vi "Facade.vi"(0 "Data In":T7, 2 "Display State In":T4, 3 "Container State":T6) -> (6 "Data Out":T7, 7 "Display State Out":T4, 8 "Action":T3)   [LabVIEW 2017, in "2D Feather.xctl"]
uses:
  <vilib>/Math Plots/2D Math Plots/2D Feather/2D Feather XCtrl/2D Feather.xctl
  <vilib>/Math Plots/2D Math Plots/2D Feather/2D Feather XCtrl/Data.ctl
  <vilib>/Math Plots/2D Math Plots/2D Plot/2D Plot Datatype/2D Plot Datatype.lvclass
  <vilib>/_xctls/Container State.ctl
  <vilib>/Math Plots/2D Math Plots/2D Feather/2D Feather XCtrl/State.ctl
  <vilib>/Math Plots/2D Math Plots/2D Feather/2D Feather/2D Feather.lvclass
  e:/builds/penguin/labview/branches/2017/dev/dist/vi.lib/Math Plots/2D Math Plots/2D Plot/2D Plot/2D Plot.lvclass
  <vilib>/Math Plots/2D Math Plots/2D Plot/Action String/2DMathPlot Ctrl Act Queue.ctl
  <vilib>/Math Plots/2D Math Plots/2D Plot/Action String/2DMathPlot Ctrl Act Cluster.ctl
  <vilib>/Math Plots/2D Math Plots/2D Plot/Action String/2DMathPlot State Class.ctl
  <vilib>/_xctls/Action.ctl
  <vilib>/Math Plots/2D Math Plots/2D Plot/2D Plot/Typedef/Range Cluster.ctl
  <vilib>/Math Plots/2D Math Plots/2D Plot/Action String/2DMathPlot Action String.ctl
  <vilib>/_xctls/XControlSupport.lvlib
  <vilib>/Math Plots/2D Math Plots/2D Plot/2D Plot/2D Plot.lvclass
panel:
  out "Floating":string
  in  "Customized Plot Legend":T1={"Color Pair Array"=[{"String"="Plot 0", "Picture"=bytes[184]}, {"String"="Plot 2", "Picture"=bytes[92]}, {"String"="Plot 3", "Picture"=bytes[92]}]}
  out "Z Axis":T2(graph)
  out "Plot Area":T2(graph)
  # "90"
  # "180"
  # "270"
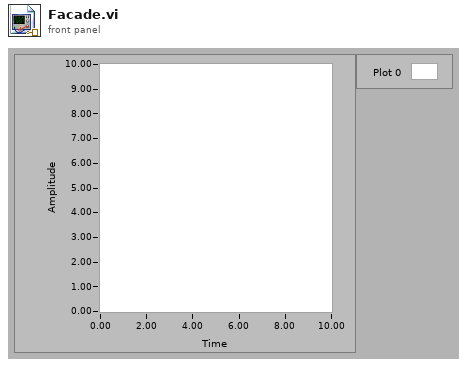
[diagram p1: front panel]
types:
  T1 = cluster{"Color Pair Array":cluster{"String":string, "Picture":picture}[]}
  T2 = cluster{"Vertex X Array":dbl[], "Vertex Y Array":dbl[]}[]
  T3 = typedef "XControlSupport.lvlib/Action.ctl" = cluster{"Data Changed?":bool, "State Changed?":bool, "Action Name":string}
  T4 = typedef "2D Feather.xctl/State.ctl" = cluster{"2D Feather.lvclass":refnum<class "2D Feather.lvclass">, "Control Ref Queue":T5, "Main Frame Color":u32, "Plot Legend Color":u32}
  T5 = typedef "2DMathPlot Ctrl Act Queue.ctl" = refnum<queue>
  T6 = typedef "XControlSupport.lvlib/Container State.ctl" = cluster{"Indicator?":bool, "Run Mode?":bool, " Refnum":refnum<vi>}
  T7 = typedef "2D Feather.xctl/Data.ctl" = refnum<class "2D Plot Datatype.lvclass">[]
  T8 = typedef "2DMathPlot Ctrl Act Cluster.ctl" = cluster{"Plot Area Ref":refnum<vi>, "Z Axis Ref":refnum<vi>, "Legend Ref":refnum<vi>, "XControl Ref":refnum<vi>, "Facade Ref":refnum<vi>, "Display State Change Class":T9}
  T9 = typedef "2DMathPlot State Class.ctl" = enum16{"Update All (Undo)", "Update General", "Update Appearance", "Update Format", "Update Scale", "Update Marker", "Update Cursor", "None"}
  T10 = typedef "2D Plot.lvclass/Range Cluster.ctl" = cluster{"X Range":cluster{"Max X":dbl, "Min X":dbl}, "Y Range":cluster{"Max Y":dbl, "Min Y":dbl}}
  T11 = typedef "2D Plot.lvclass/Multiplot Representation.ctl" = cluster{"Plot Representation Array":T12[], "Max Range":T10}
  T12 = typedef "2D Plot.lvclass/Plot Representation.ctl" = cluster{"Plot Range":T10, "Vertex Cluster":cluster{"Vertex X Array":dbl[], "Vertex Y Array":dbl[]}, "Base Cluster":cluster{"Base X Array":dbl[], "Base Y Array":dbl[]}}
  T13 = typedef "2DMathPlot Action String.ctl" = u16
  T14 = typedef "LVPoint32TypeDef.ctl" = cluster{"Horizontal":i32, "Vertical":i32}
  T15 = typedef "LVRectTypeDef.ctl" = cluster{"Left":i16, "Top":i16, "Right":i16, "Bottom":i16}
  T16 = typedef "LVRangeTypeDef.ctl" = cluster{"Minimum":dbl, "Maximum":dbl, "Increment":dbl, "Minor Increment":dbl, "Start":dbl}
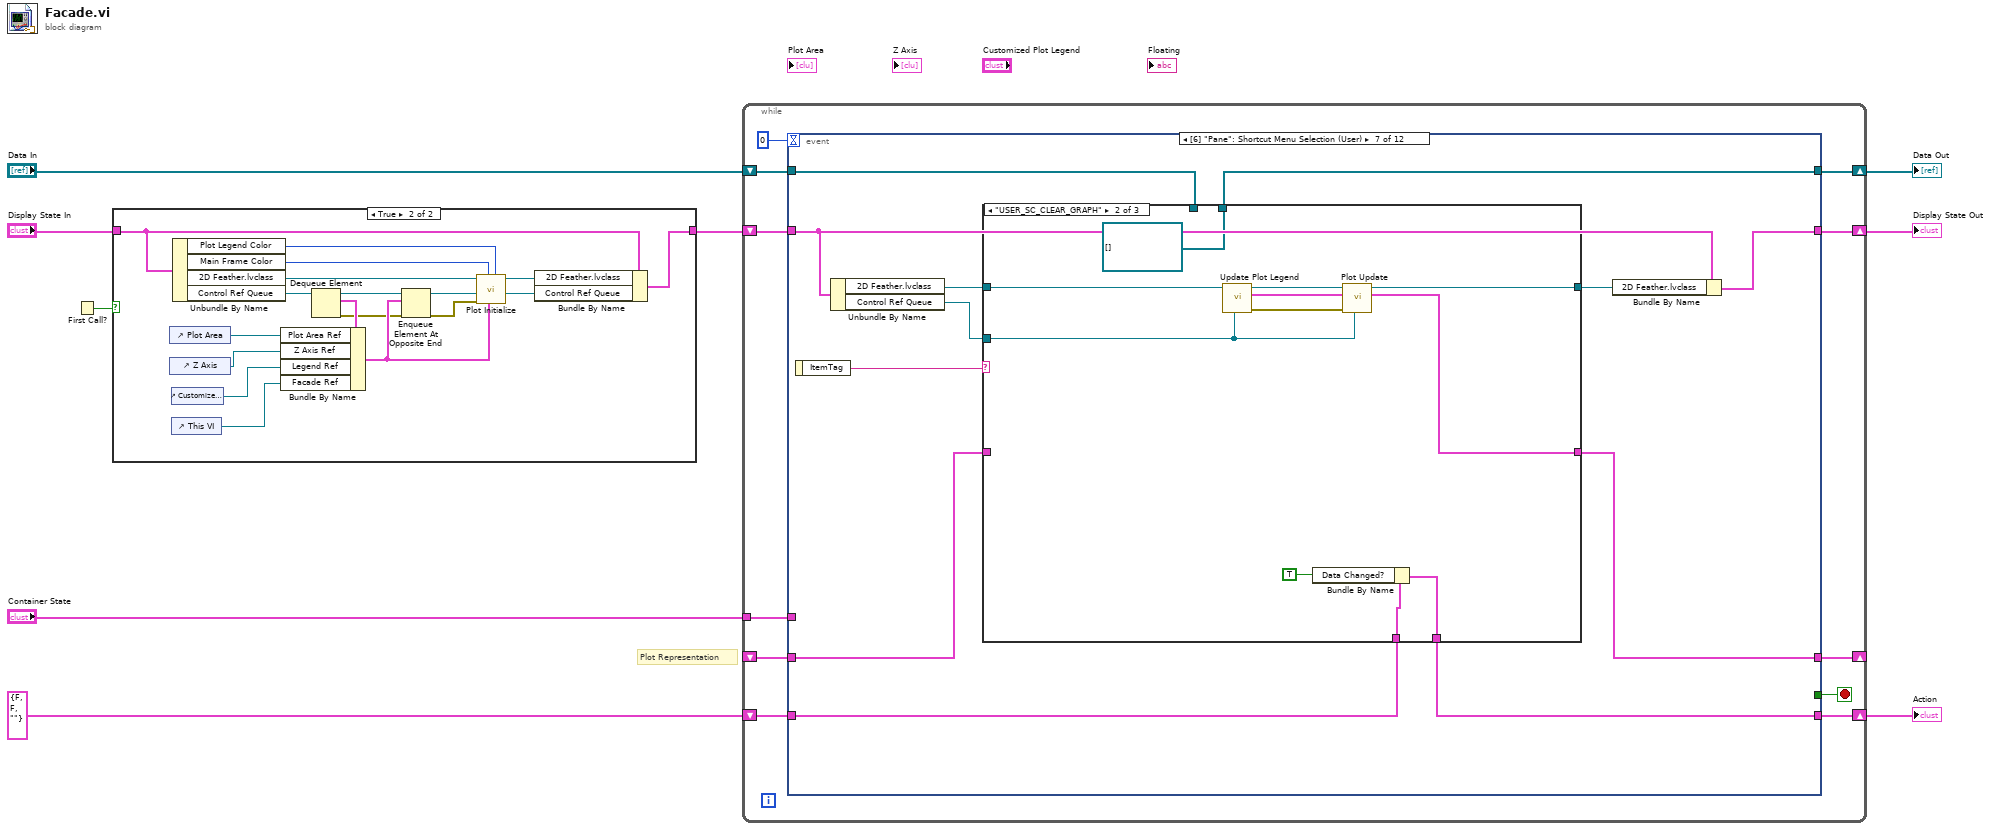
[diagram p0: block diagram]
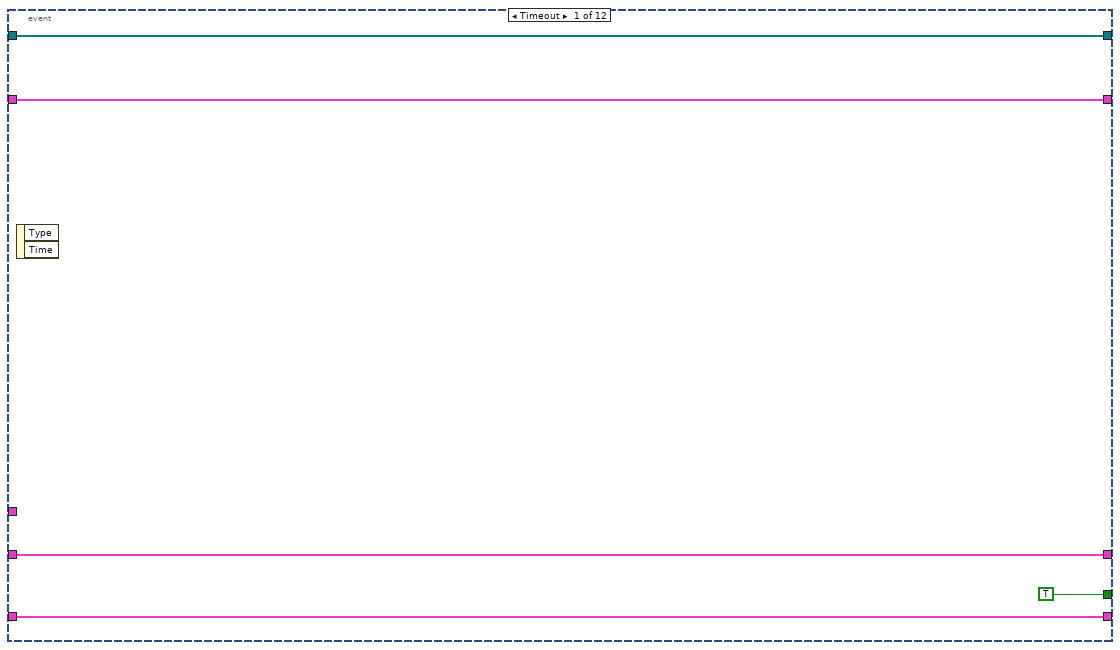
[diagram p3: hidden frame]
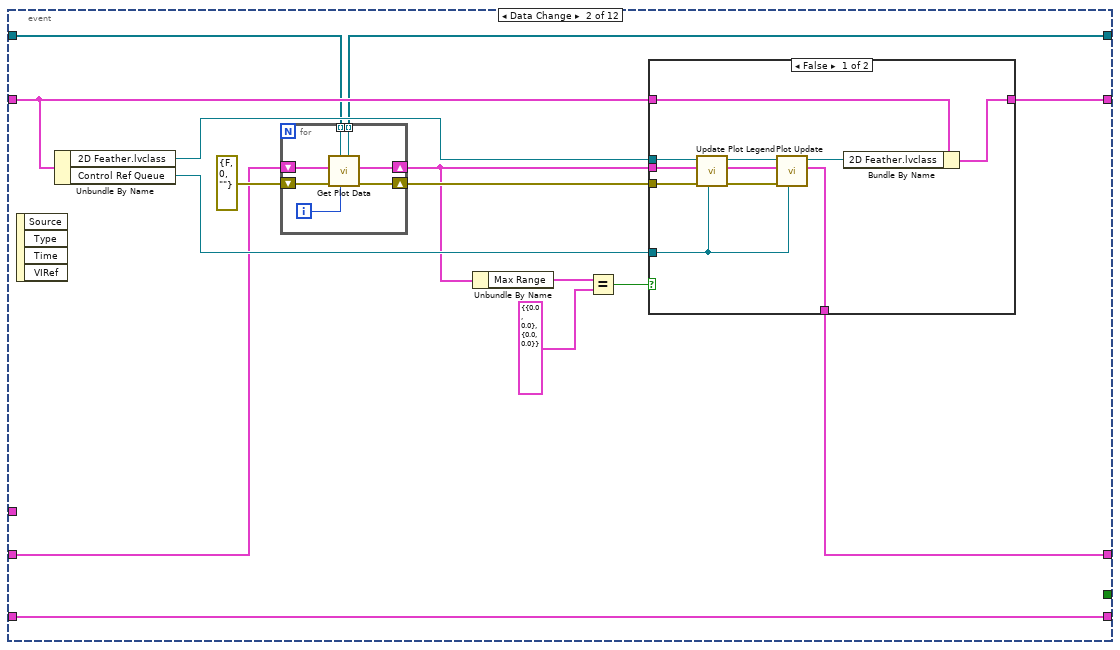
[diagram p4: hidden frame]
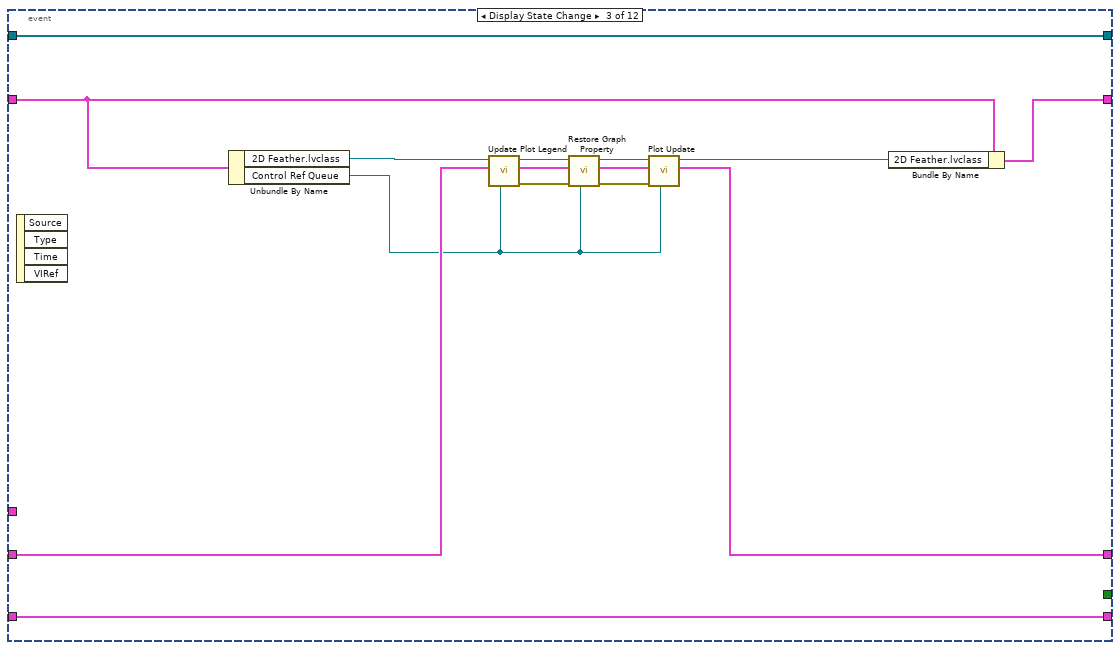
[diagram p6: hidden frame]
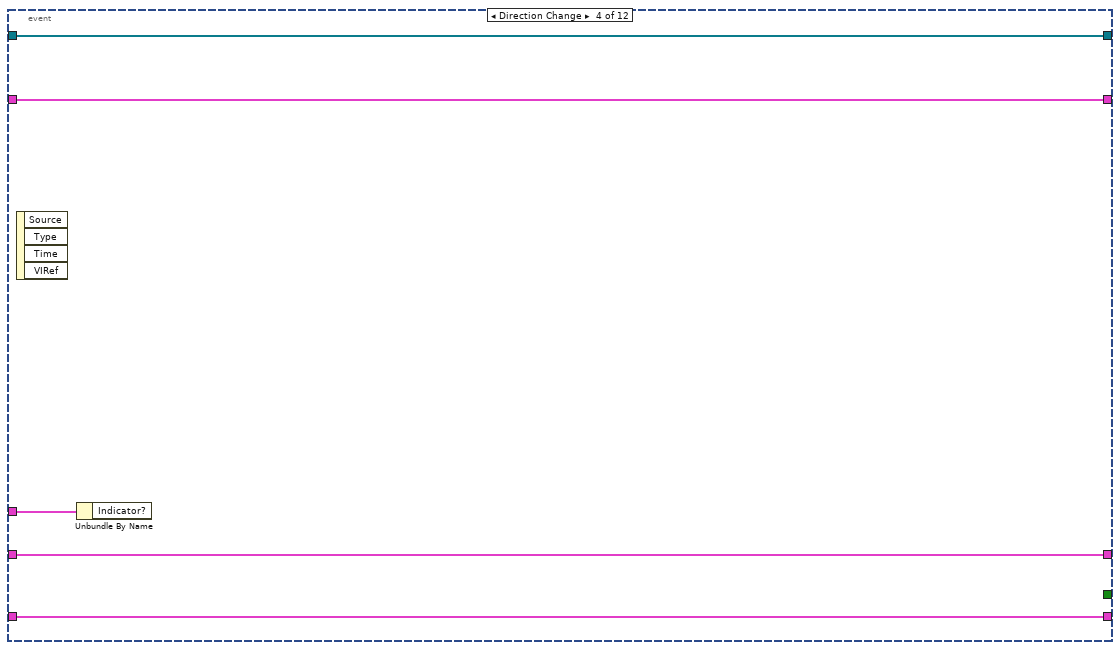
[diagram p7: hidden frame]
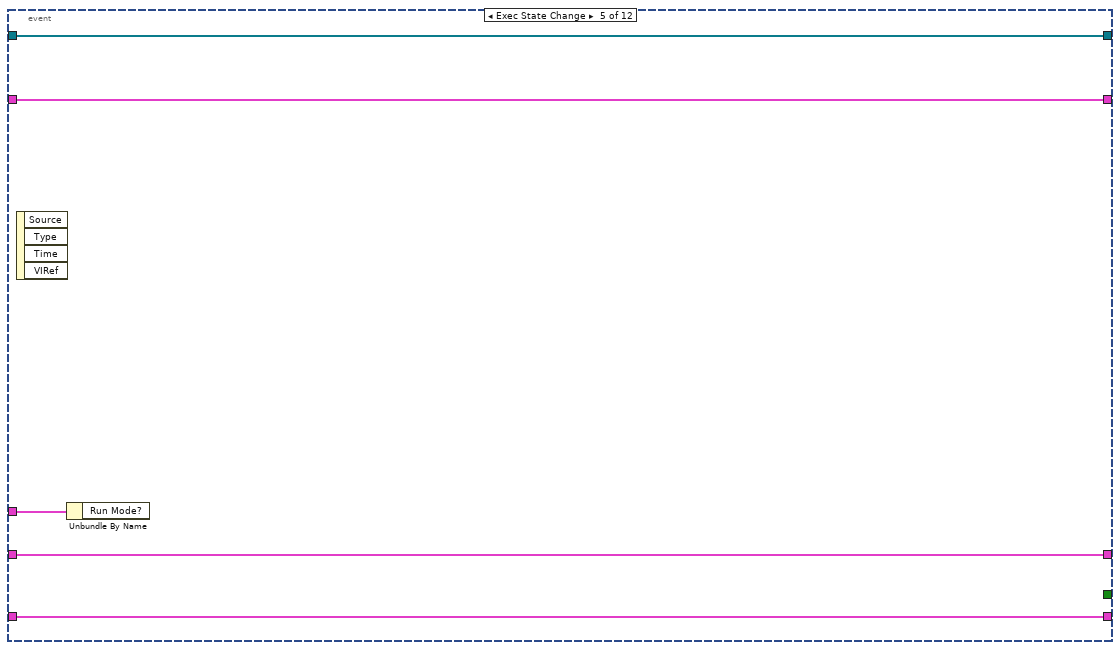
[diagram p8: hidden frame]
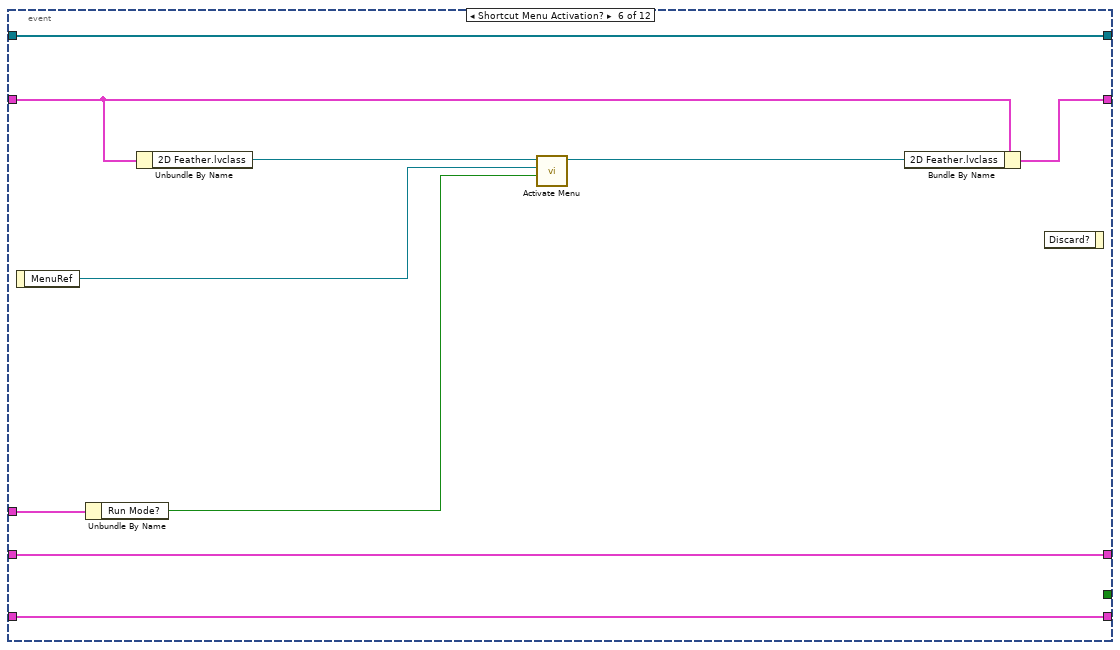
[diagram p9: hidden frame]
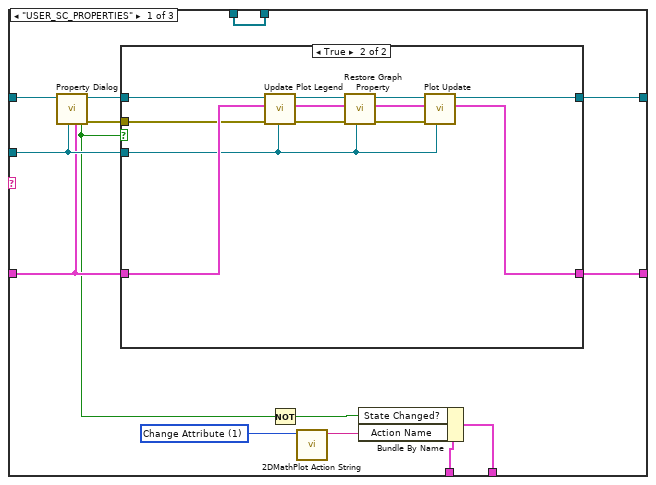
[diagram p10: hidden frame]
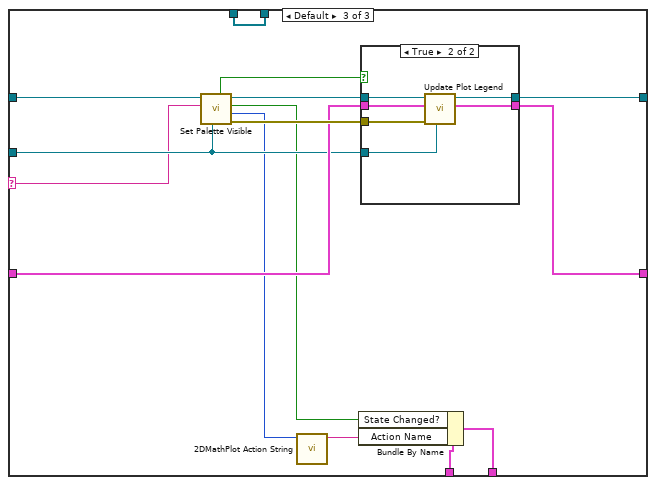
[diagram p12: hidden frame]
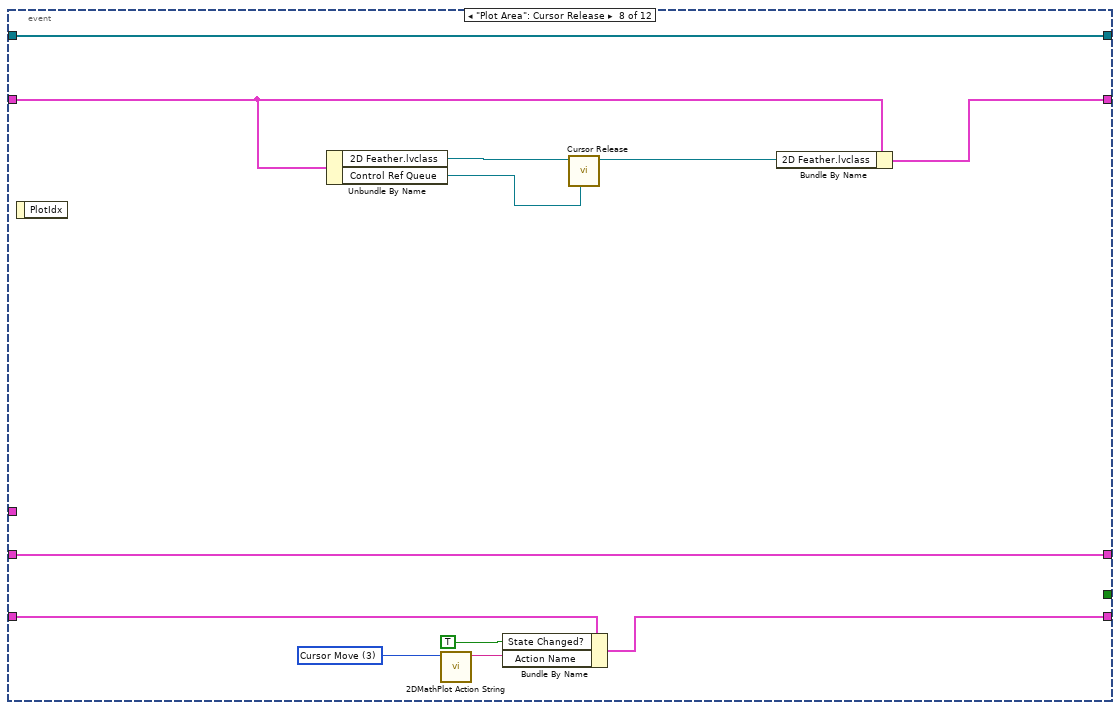
[diagram p14: hidden frame]
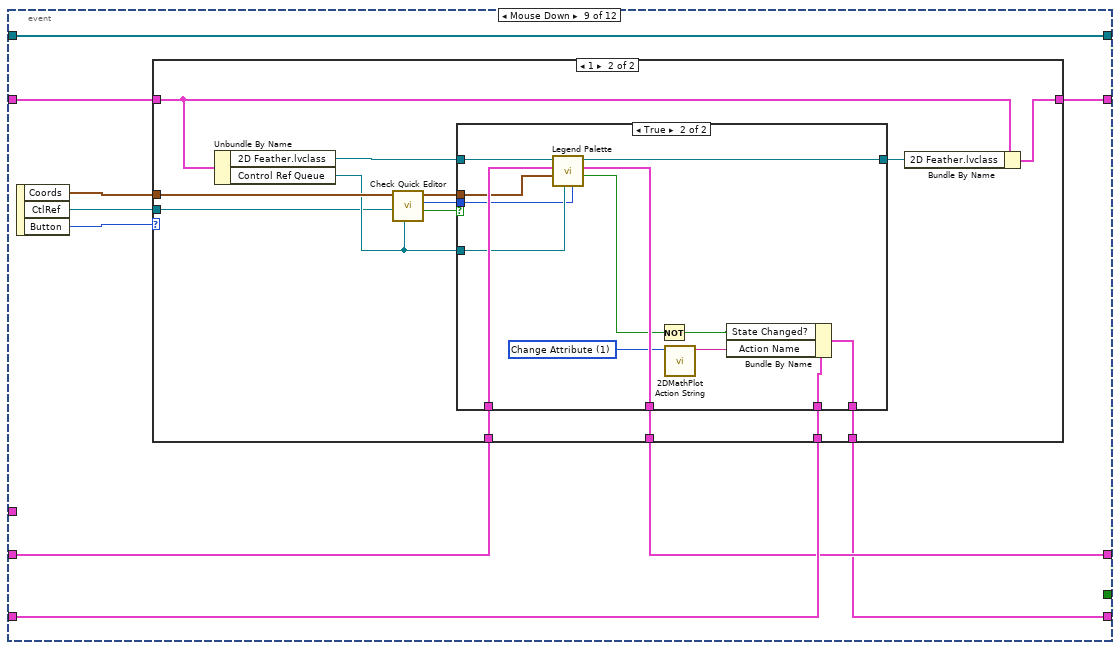
[diagram p15: hidden frame]
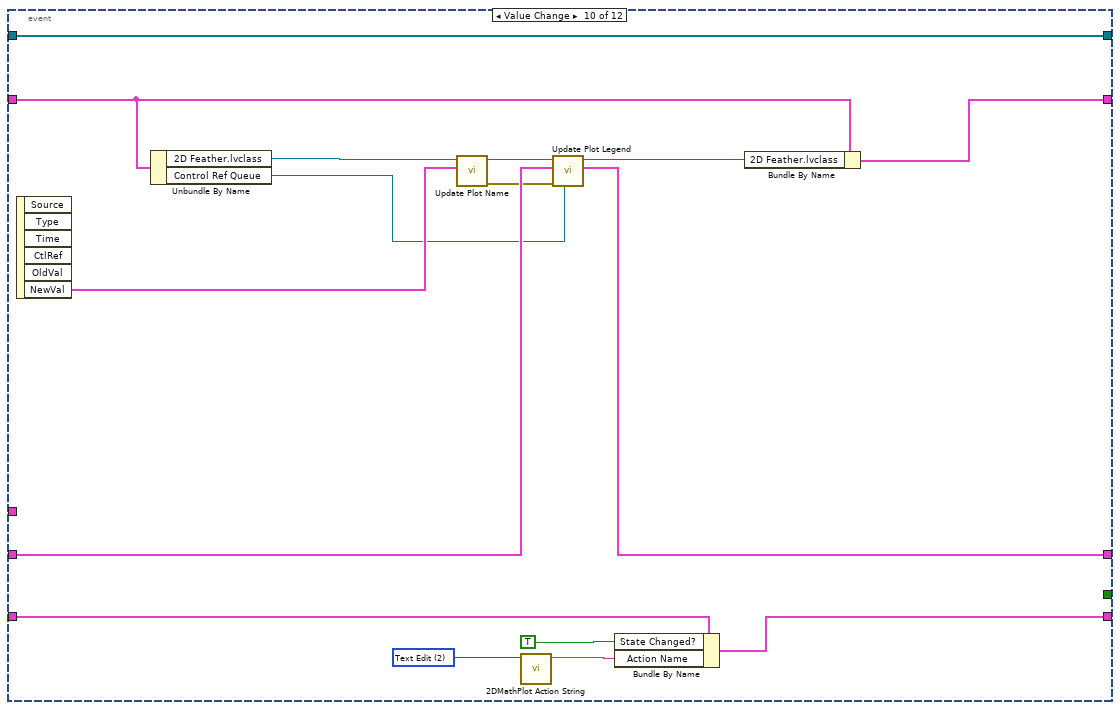
[diagram p18: hidden frame]
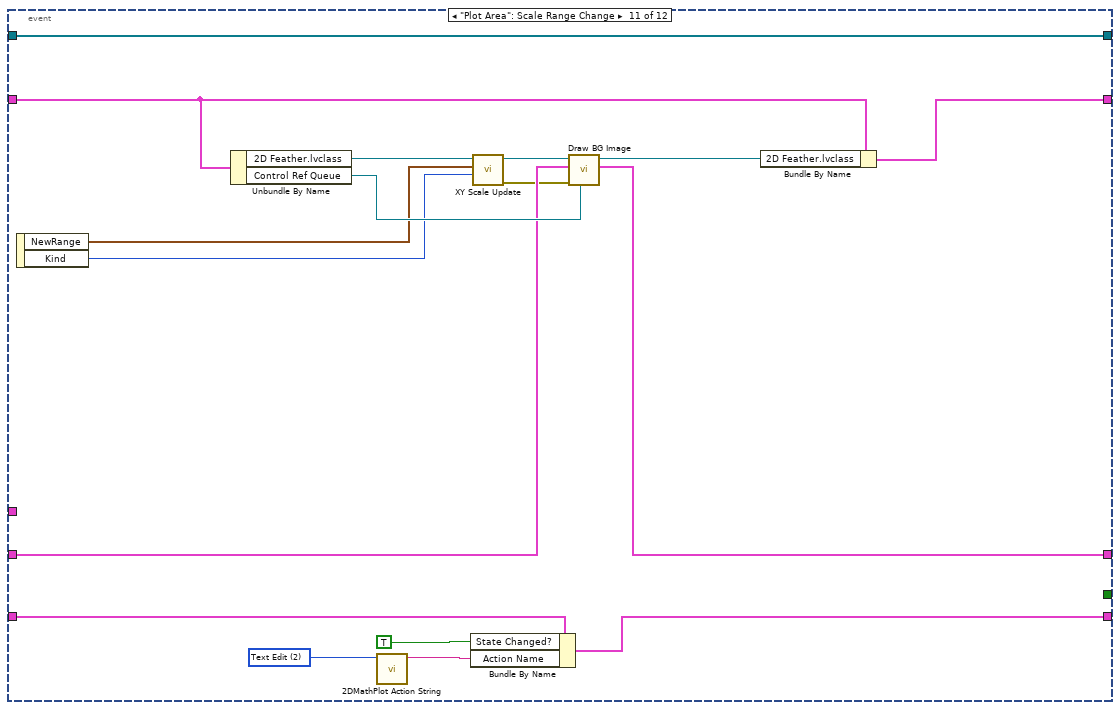
[diagram p19: hidden frame]
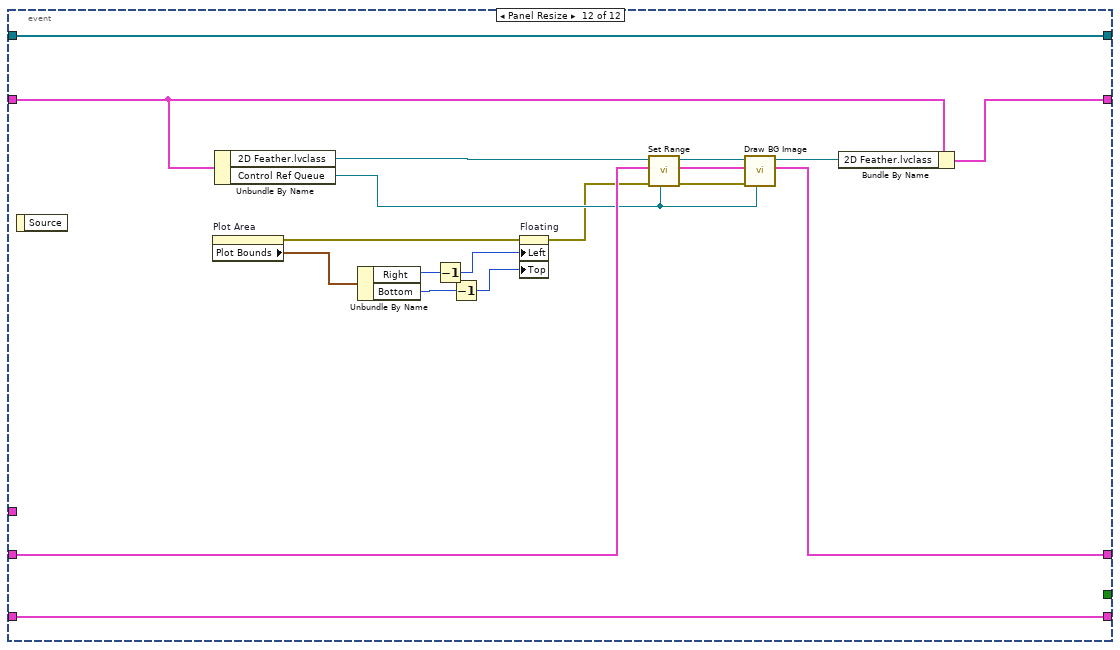
[diagram p20: hidden frame]
diagram:
  # "Plot Representation"
  n1 = First Call?() -> (First Call?: T/F=w3:bool)
  n2 = case shown="True" w3 {
    tunnel: "Display State In" -> [w10 w17]
    tunnel: [w10 w16] -> w1
    frame False {
    }
    frame True {
      n3 = control-ref of="Plot Area"() -> (w15:refnum<vi>)
      n4 = control-ref of="Z Axis"() -> (w24:refnum<vi>)
      n5 = control-ref of="Customized Plot Legend"() -> (w14:refnum<vi>)
      n6 = control-ref of="This VI"() -> (w13:refnum<vi>)
      n7 = Unbundle By Name(w17) -> ("Plot Legend Color"=w11:u32, "Main Frame Color"=w12:u32, "2D Feather.lvclass"=w23:refnum<class "2D Feather.lvclass">, "Control Ref Queue"=w27:T5)
      n8 = Dequeue Element(queue=w27) -> (queue out=w26:T5, element=w25:T8, error out=w20:errorcluster)  [unwired: 1 in, 2 out]
      n9 = Bundle By Name(cluster=w25, "Plot Area Ref"=w15, "Z Axis Ref"=w24, "Legend Ref"=w14, "Facade Ref"=w13) -> (w22:T8)
      n10 = Enqueue Element At Opposite End(queue=w26, element=w22, error in (no error)=w20) -> (queue out=w18:T5, error out=w21:errorcluster)  [unwired: 2 out]
      n11 = call-dynamic "Plot Initialize.vi"("Plot Legend Color"=w11, "Control Ref Cluster"=w22, "Main Frame Color"=w12, "error in (no error)"=w21, "2D Plot.lvclass in"=w23) -> ("2D Plot.lvclass out"=w19:refnum<class "2D Feather.lvclass">)  [unwired: 6 out]
      n12 = Bundle By Name(cluster=w17, "2D Feather.lvclass"=w19, "Control Ref Queue"=w18) -> (w16:T4)
    }
  }
  n13 = while {
    shift-right: [w37] -> w6
    shift-left: w1 -> [w38]
    tunnel: "Container State" -> [w34]
    shift-right: [w32] -> w9
    shift-left: "Data In" -> [w33]
    shift-right: [w30] -> w5
    shift-left: T3 {"Data Changed?"=FALSE, "State Changed?"=FALSE, "Action Name"=""} ("Action") -> [w31]
    shift-right: [w28] -> _
    shift-left: _ -> [w29]
    stop <- w36 stop-if-true
    n14 = event shown="[6] \"Pane\": Shortcut Menu Selection (User)" {
      selector: _ -> [_ _ _ _ _ _ _ _ _ _ _ _]
      dyn-events: _ -> [_ _ _ _ _ _ _ _ _ _ _ _]
      timeout: 0 -> [_ _ _ _ _ _ _ _ _ _ _ _]
      tunnel: w38 -> [w40 w49 w91 w96 w101 w106 w124 w193 w207 w254 w266 w290]
      tunnel: [w40 w46 w90 w96 w101 w105 w123 w192 w205 w255 w265 w289] -> w37
      tunnel: [TRUE _ _ _ _ _ _ _ _ _ _ _] -> w36
      tunnel: w34 -> [_ _ _ w97 w102 w111 _ _ _ _ _ _]
      tunnel: w33 -> [w41 w48 w89 w95 w100 w112 w114 w197 w206 w256 w273 w292]
      tunnel: [w41 w47 w89 w95 w100 w112 w113 w197 w206 w256 w273 w292] -> w32
      tunnel: [w42 w44 w92 w94 w99 w103 w117 w195 w198 w249 w271 w291] -> w30
      tunnel: w31 -> [w42 w44 w92 w94 w99 w103 w116 w196 w200 w250 w272 w291]
      tunnel: w29 -> [w39 w50 w84 w93 w98 w104 w118 w194 w201 w244 w263 w283]
      tunnel: [w39 w45 w79 w93 w98 w104 w115 w194 w199 w243 w262 w287] -> w28
      event Timeout {
        n15 = event-data() -> ()  [unwired: 3 out]
      }
      event Data Change {
        n16 = event-data() -> ()  [unwired: 5 out]
        n17 = Unbundle By Name(w49) -> ("2D Feather.lvclass"=w57:refnum<class "2D Feather.lvclass">, "Control Ref Queue"=w56:T5)
        n18 = for {
          tunnel: w48 -> [w75] mode=indexing
          tunnel: [w74] -> w47 mode=indexing
          shift-right: [w76] -> w55
          shift-left: errorcluster {"status"=FALSE, "code"=0, "source"=""} ("error out") -> [w72]
          shift-right: [w77] -> w52
          shift-left: w50 -> [w78]
          i -> [w73]
          n19 = call <vilib>:"Get Plot Data.vi"("Index"=w73, "2D Plot Datatype.lvclass in"=w75, "error in (no error)"=w72, "Multiplot Representation In"=w78) -> ("error out"=w76:errorcluster, "Multiplot Representation Out"=w77:T11, "2D Plot Datatype.lvclass out"=w74:refnum<class "2D Plot Datatype.lvclass">)  [unwired: 5 out]
        }
        n20 = Unbundle By Name(w52) -> ("Max Range"=w53:T10)
        n21 = Equal?(x=w53, y=T10 {"X Range"={"Max X"=0.0, "Min X"=0.0}, "Y Range"={"Max Y"=0.0, "Min Y"=0.0}} ("Max Range")) -> (x = y?=w51:bool)
        n22 = case shown="False" w51 {
          tunnel: w49 -> [w69 w70]
          tunnel: [w68 w70] -> w46
          tunnel: [w66 w71] -> w45
          tunnel: w57 -> [w65 _]
          tunnel: w52 -> [w63 w71]
          tunnel: w56 -> [w61 _]
          tunnel: w55 -> [w60 _]
          frame False {
            n23 = call <vilib>:"Update Plot Legend.vi"("Control Ref Queue"=w61, "error in (no error)"=w60, "Multiplot Representation In"=w63, "2D Plot in"=w65) -> ("error out"=w59:errorcluster, "Multiplot Representation Out"=w62:T11, "2D Plot out"=w64:refnum<class "2D Feather.lvclass">)  [unwired: 5 out]
            n24 = call <vilib>:"Plot Update.vi"("Control Ref Queue"=w61, "error in (no error)"=w59, "Multiplot Representation In"=w62, "2D Plot.lvclass in"=w64) -> ("Multiplot Representation Out"=w66:T11, "2D Plot.lvclass out"=w67:refnum<class "2D Feather.lvclass">)  [unwired: 6 out]
            n25 = Bundle By Name(cluster=w69, "2D Feather.lvclass"=w67) -> (w68:T4)
          }
          frame True {
          }
        }
      }
      event Display State Change {
        n26 = event-data() -> ()  [unwired: 5 out]
        n27 = Unbundle By Name(w91) -> ("2D Feather.lvclass"=w86:refnum<class "2D Feather.lvclass">, "Control Ref Queue"=w82:T5)
        n28 = call <vilib>:"Update Plot Legend.vi"("Control Ref Queue"=w82, "Multiplot Representation In"=w84, "2D Plot in"=w86) -> ("error out"=w83:errorcluster, "Multiplot Representation Out"=w80:T11, "2D Plot out"=w85:refnum<class "2D Feather.lvclass">)  [unwired: 1 in, 5 out]
        n29 = call-dynamic "Restore Graph Property.vi"("Control Ref Queue"=w82, "error in (no error)"=w83, "2D Plot.lvclass in"=w85) -> ("error out"=w81:errorcluster, "2D Plot.lvclass out"=w88:refnum<class "2D Feather.lvclass">)  [unwired: 1 in, 6 out]
        n30 = call <vilib>:"Plot Update.vi"("Control Ref Queue"=w82, "error in (no error)"=w81, "Multiplot Representation In"=w80, "2D Plot.lvclass in"=w88) -> ("Multiplot Representation Out"=w79:T11, "2D Plot.lvclass out"=w87:refnum<class "2D Feather.lvclass">)  [unwired: 6 out]
        n31 = Bundle By Name(cluster=w91, "2D Feather.lvclass"=w87) -> (w90:T4)
      }
      event Direction Change {
        n32 = event-data() -> ()  [unwired: 5 out]
        n33 = Unbundle By Name(w97) -> ()  [unwired: 1 out]
      }
      event Exec State Change {
        n34 = event-data() -> ()  [unwired: 5 out]
        n35 = Unbundle By Name(w102) -> ()  [unwired: 1 out]
      }
      event Shortcut Menu Activation? {
        n36 = event-data() -> ("MenuRef"=w110:refnum<k9>)  [unwired: 1 out]
        n37 = Unbundle By Name(w111) -> ("Run Mode?"=w109:bool)
        n38 = Unbundle By Name(w106) -> ("2D Feather.lvclass"=w108:refnum<class "2D Feather.lvclass">)
        n39 = call-dynamic "Activate Menu.vi"("Run mode?"=w109, "MenuRef"=w110, "2D Plot.lvclass in"=w108) -> ("2D Plot.lvclass out"=w107:refnum<class "2D Feather.lvclass">)  [unwired: 1 in, 7 out]
        n40 = Bundle By Name(cluster=w106, "2D Feather.lvclass"=w107) -> (w105:T4)
        n41 = event-data() -> ()  [unwired: 1 in, 2 out]
      }
      event Shortcut Menu Selection (User) {
        n42 = event-data() -> ("ItemTag"=w119:string)  [unwired: 1 out]
        n43 = Unbundle By Name(w124) -> ("2D Feather.lvclass"=w122:refnum<class "2D Feather.lvclass">, "Control Ref Queue"=w120:T5)
        n44 = case shown="\"USER_SC_CLEAR_GRAPH\"" w119 {
          selector: w119 -> [_ _ w166]
          tunnel: [w136 w156 w169] -> w121
          tunnel: w122 -> [w138 w158 w177]
          tunnel: w120 -> [w135 w157 w170]
          tunnel: w118 -> [w134 _ w172]
          tunnel: [w128 w153 w176] -> w117
          tunnel: w116 -> [w129 w154 w175]
          tunnel: [w133 w155 w168] -> w115
          tunnel: [w125 T7 [] ("Data") w167] -> w113
          tunnel: w114 -> [w125 _ w167]
          frame "USER_SC_PROPERTIES" {
            w131 = T13 1 items=["Show/Hide", "Change Attribute", "Text Edit", "Cursor Move"] ("Global String")
            n45 = call-dynamic "Property Dialog.vi"("Control Ref Queue"=w135, "Multiplot Representation"=w134, "2D Feather.lvclass in"=w138) -> ("error out"=w132:errorcluster, "2D Feather.lvclass out"=w137:refnum<class "2D Feather.lvclass">, "Cancel?"=w127:bool)  [unwired: 1 in, 5 out]
            n46 = case shown="True" w127 {
              tunnel: w137 -> [w140 w149]
              tunnel: [w140 w145] -> w136
              tunnel: w135 -> [_ w141]
              tunnel: w134 -> [w139 w151]
              tunnel: [w139 w142] -> w133
              tunnel: w132 -> [_ w148]
              frame False {
              }
              frame True {
                n47 = call <vilib>:"Update Plot Legend.vi"("Control Ref Queue"=w141, "error in (no error)"=w148, "Multiplot Representation In"=w151, "2D Plot in"=w149) -> ("error out"=w147:errorcluster, "Multiplot Representation Out"=w143:T11, "2D Plot out"=w150:refnum<class "2D Feather.lvclass">)  [unwired: 5 out]
                n48 = call-dynamic "Restore Graph Property.vi"("Control Ref Queue"=w141, "error in (no error)"=w147, "2D Plot.lvclass in"=w150) -> ("error out"=w144:errorcluster, "2D Plot.lvclass out"=w146:refnum<class "2D Feather.lvclass">)  [unwired: 1 in, 6 out]
                n49 = call <vilib>:"Plot Update.vi"("Control Ref Queue"=w141, "error in (no error)"=w144, "Multiplot Representation In"=w143, "2D Plot.lvclass in"=w146) -> ("Multiplot Representation Out"=w142:T11, "2D Plot.lvclass out"=w145:refnum<class "2D Feather.lvclass">)  [unwired: 6 out]
              }
            }
            n50 = Not(x=w127) -> (.not. x?=w126:bool)
            n51 = call <vilib>:"2DMathPlot Action String.vi"("Global String"=w131) -> ("String Out"=w130:string)  [unwired: 10 out]
            n52 = Bundle By Name(cluster=w129, "State Changed?"=w126, "Action Name"=w130) -> (w128:T3)
          }
          frame "USER_SC_CLEAR_GRAPH" {
            n53 = call <vilib>:"Update Plot Legend.vi"("Control Ref Queue"=w157, "2D Plot in"=w158) -> ("error out"=w160:errorcluster, "Multiplot Representation Out"=w161:T11, "2D Plot out"=w162:refnum<class "2D Feather.lvclass">)  [unwired: 2 in, 5 out]
            n54 = Bundle By Name(cluster=w154, "Data Changed?"=TRUE) -> (w153:T3)
            n55 = call <vilib>:"Plot Update.vi"("Control Ref Queue"=w157, "error in (no error)"=w160, "Multiplot Representation In"=w161, "2D Plot.lvclass in"=w162) -> ("Multiplot Representation Out"=w155:T11, "2D Plot.lvclass out"=w156:refnum<class "2D Feather.lvclass">)  [unwired: 6 out]
          }
          frame Default {
            n56 = call-dynamic "Set Palette Visible.vi"("Control Ref Queue"=w170, "Item Tag"=w166, "2D Plot in"=w177) -> ("error out"=w173:errorcluster, "Action String"=w163:T13, "State Change?"=w164:bool, "2D Plot out"=w171:refnum<class "2D Feather.lvclass">, "Update Legend?"=w165:bool)  [unwired: 2 in, 2 out]
            n57 = call <vilib>:"2DMathPlot Action String.vi"("Global String"=w163) -> ("String Out"=w174:string)  [unwired: 10 out]
            n58 = Bundle By Name(cluster=w175, "State Changed?"=w164, "Action Name"=w174) -> (w176:T3)
            n59 = case shown="True" w165 {
              tunnel: w171 -> [w179 w185]
              tunnel: [w179 w184] -> w169
              tunnel: w172 -> [w178 w183]
              tunnel: [w178 w182] -> w168
              tunnel: w173 -> [_ w181]
              tunnel: w170 -> [_ w180]
              frame False {
              }
              frame True {
                n60 = call <vilib>:"Update Plot Legend.vi"("Control Ref Queue"=w180, "error in (no error)"=w181, "Multiplot Representation In"=w183, "2D Plot in"=w185) -> ("Multiplot Representation Out"=w182:T11, "2D Plot out"=w184:refnum<class "2D Feather.lvclass">)  [unwired: 6 out]
              }
            }
          }
        }
        n61 = Bundle By Name(cluster=w124, "2D Feather.lvclass"=w121) -> (w123:T4)
      }
      event "Plot Area": Cursor Release {
        w187 = T13 3 items=["Show/Hide", "Change Attribute", "Text Edit", "Cursor Move"] ("Global String")
        n62 = event-data() -> ()  [unwired: 2 out]
        n63 = Unbundle By Name(w193) -> ("2D Feather.lvclass"=w191:refnum<class "2D Feather.lvclass">, "Control Ref Queue"=w186:T5)
        n64 = call <vilib>:"2DMathPlot Action String.vi"("Global String"=w187) -> ("String Out"=w188:string)  [unwired: 10 out]
        n65 = Bundle By Name(cluster=w196, "State Changed?"=TRUE, "Action Name"=w188) -> (w195:T3)
        n66 = call <vilib>:"Cursor Release.vi"("Control Ref Queue"=w186, "2D Plot.lvclass in"=w191) -> ("2D Plot.lvclass out"=w190:refnum<class "2D Feather.lvclass">)  [unwired: 1 in, 8 out]
        n67 = Bundle By Name(cluster=w193, "2D Feather.lvclass"=w190) -> (w192:T4)
      }
      event "Customized Plot Legend.Color Pair Array": Mouse Down {
        n68 = event-data() -> ("Coords"=w204:T14, "CtlRef"=w203:refnum<vi>, "Button"=w202:u16)  [unwired: 1 out]
        n69 = case shown="1" w202 {
          tunnel: w207 -> [w208 w222]
          tunnel: [w208 w221] -> w205
          tunnel: w201 -> [w210 w220]
          tunnel: [w210 w219] -> w199
          tunnel: w200 -> [w209 w218]
          tunnel: [w209 w217] -> w198
          tunnel: w204 -> [_ w216]
          tunnel: w203 -> [_ w214]
          frame Default {
          }
          frame 1 {
            n70 = Unbundle By Name(w222) -> ("2D Feather.lvclass"=w224:refnum<class "2D Feather.lvclass">, "Control Ref Queue"=w215:T5)
            n71 = call <vilib>:"Check Quick Editor.vi"("Control Ref Queue"=w215, "Array Element"=w214, "Coords"=w216) -> ("Pop?"=w213:bool, "Active Plot"=w211:i32, "Window Bounds"=w212:T15)  [unwired: 1 in, 5 out]
            n72 = case shown="True" w213 {
              tunnel: w224 -> [w227 w240]
              tunnel: [w227 w239] -> w223
              tunnel: w220 -> [w226 w238]
              tunnel: [w226 w237] -> w219
              tunnel: w218 -> [w225 w236]
              tunnel: [w225 w235] -> w217
              tunnel: w215 -> [_ w230]
              tunnel: w212 -> [_ w229]
              tunnel: w211 -> [_ w228]
              frame False {
              }
              frame True {
                w234 = T13 1 items=["Show/Hide", "Change Attribute", "Text Edit", "Cursor Move"] ("Global String")
                n73 = call-dynamic "Legend Palette.vi"("Active Plot"=w228, "Control Ref Queue"=w230, "Window Bounds"=w229, "Multiplot Representation In"=w238, "2D Feather.lvclass in"=w240) -> ("Cancel?"=w232:bool, "Multiplot Representation Out"=w237:T11, "2D Feather.lvclass out"=w239:refnum<class "2D Feather.lvclass">)  [unwired: 4 out]
                n74 = Not(x=w232) -> (.not. x?=w231:bool)
                n75 = call <vilib>:"2DMathPlot Action String.vi"("Global String"=w234) -> ("String Out"=w233:string)  [unwired: 10 out]
                n76 = Bundle By Name(cluster=w236, "State Changed?"=w231, "Action Name"=w233) -> (w235:T3)
              }
            }
            n77 = Bundle By Name(cluster=w222, "2D Feather.lvclass"=w223) -> (w221:T4)
          }
        }
      }
      event "Customized Plot Legend.Color Pair Array": Value Change {
        w252 = T13 2 items=["Show/Hide", "Change Attribute", "Text Edit", "Cursor Move"] ("Global String")
        n78 = event-data() -> ("NewVal"=w248:cluster{"String":string, "Picture":picture}[])  [unwired: 6 out]
        n79 = Unbundle By Name(w254) -> ("2D Feather.lvclass"=w247:refnum<class "2D Feather.lvclass">, "Control Ref Queue"=w241:T5)
        n80 = call-dynamic "Update Plot Name.vi"("NewVal"=w248, "2D Feather.lvclass in"=w247) -> ("error out"=w242:errorcluster, "2D Feather.lvclass out"=w246:refnum<class "2D Feather.lvclass">)  [unwired: 2 in, 6 out]
        n81 = call <vilib>:"2DMathPlot Action String.vi"("Global String"=w252) -> ("String Out"=w253:string)  [unwired: 10 out]
        n82 = call <vilib>:"Update Plot Legend.vi"("Control Ref Queue"=w241, "error in (no error)"=w242, "Multiplot Representation In"=w244, "2D Plot in"=w246) -> ("Multiplot Representation Out"=w243:T11, "2D Plot out"=w245:refnum<class "2D Feather.lvclass">)  [unwired: 6 out]
        n83 = Bundle By Name(cluster=w250, "State Changed?"=TRUE, "Action Name"=w253) -> (w249:T3)
        n84 = Bundle By Name(cluster=w254, "2D Feather.lvclass"=w245) -> (w255:T4)
      }
      event "Plot Area": Scale Range Change {
        w269 = T13 2 items=["Show/Hide", "Change Attribute", "Text Edit", "Cursor Move"] ("Global String")
        n85 = event-data() -> ("NewRange"=w260:T16, "Kind"=w259:enum16{"X-Scale", "Y-Scale", "Z-Scale"})  [unwired: 1 out]
        n86 = Unbundle By Name(w266) -> ("2D Feather.lvclass"=w261:refnum<class "2D Feather.lvclass">, "Control Ref Queue"=w264:T5)
        n87 = call <vilib>:"2DMathPlot Action String.vi"("Global String"=w269) -> ("String Out"=w270:string)  [unwired: 10 out]
        n88 = Bundle By Name(cluster=w272, "State Changed?"=TRUE, "Action Name"=w270) -> (w271:T3)
        n89 = call <vilib>:"XY Scale Update.vi"("Kind"=w259, "NewRange"=w260, "2D Plot.lvclass in"=w261) -> ("error out"=w257:errorcluster, "2D Plot.lvclass out"=w258:refnum<class "2D Feather.lvclass">)  [unwired: 7 in]
        n90 = call-dynamic "Draw BG Image.vi"("Control Ref Queue"=w264, "error in (no error)"=w257, "Multiplot Representation In"=w263, "2D Feather.lvclass in"=w258) -> ("Multiplot Representation Out"=w262:T11, "2D Feather.lvclass out"=w267:refnum<class "2D Feather.lvclass">)  [unwired: 6 out]
        n91 = Bundle By Name(cluster=w266, "2D Feather.lvclass"=w267) -> (w265:T4)
      }
      event Panel Resize {
        n92 = event-data() -> ()  [unwired: 2 out]
        n93 = property on="Plot Area" class="XYGraph (strict)"() -> (error out=w275:errorcluster, "Plot Bounds"=w276:T15)  [unwired: 2 in, 1 out]
        n94 = Unbundle By Name(w290) -> ("2D Feather.lvclass"=w286:refnum<class "2D Feather.lvclass">, "Control Ref Queue"=w281:T5)
        n95 = Unbundle By Name(w276) -> ("Right"=w277:i16, "Bottom"=w278:i16)
        n96 = Decrement(x=w277) -> (x-1=w279:i16)
        n97 = Decrement(x=w278) -> (x-1=w280:i16)
        n98 = property on="Floating" class="Str"(error in=w275, "Left"=w279, "Top"=w280) -> (error out=w274:errorcluster)  [unwired: 1 in, 1 out]
        n99 = call-dynamic "Set Range.vi"("Control Ref Queue"=w281, "error in (no error)"=w274, "Multiplot Representation In"=w283, "2D Plot.lvclass in"=w286) -> ("error out"=w282:errorcluster, "Multiplot Representation Out"=w284:T11, "2D Plot.lvclass out"=w285:refnum<class "2D Feather.lvclass">)  [unwired: 1 in, 4 out]
        n100 = call-dynamic "Draw BG Image.vi"("Control Ref Queue"=w281, "error in (no error)"=w282, "Multiplot Representation In"=w284, "2D Feather.lvclass in"=w285) -> ("Multiplot Representation Out"=w287:T11, "2D Feather.lvclass out"=w288:refnum<class "2D Feather.lvclass">)  [unwired: 6 out]
        n101 = Bundle By Name(cluster=w290, "2D Feather.lvclass"=w288) -> (w289:T4)
      }
    }
  }
  "Display State Out" <- w6
  "Data Out" <- w9
  "Action" <- w5
